vi "64x128OLED_SSD1315YellowBlue.vi"() -> ()   [LabVIEW 2024]
uses:
  Driver/Public/Digital Pull Direction.ctl
  a7562c57-8a3f-42dc-a248-a218528d61d2.vi
  526a81f8-07e3-4dc8-9390-ead75d1578b4.vi
  Public/InitialiseOLED.vi
  Public/GetPicture.vi
  Public/BuildMessagesFromPicture.vi
  Driver/CTIPicoVISA.lvlib
  OLEDI2CMessageGenerator.lvlib
panel:
  in  "Blue 3":string="Blue3"
  in  "Blue 2":string="Blue2"
  in  "Blue 1":string="Blue1"
  in  "Yellow":string="Yellow"
  out "Numeric":i32
  in  "stop":bool
  out "2D Picture":picture
  in  "Grove Connector":enum16{"I2C0", "I2C1"}(ring)
  out "Identity":T1
  out "error out":errorcluster
  in  "Port":refnum<visa-resource-name>="COM7"
  # "https://wiki.seeedstudio.com/Grove-OLED-Yellow&Blue-Display-0.96-SSD1315_V1.0/"
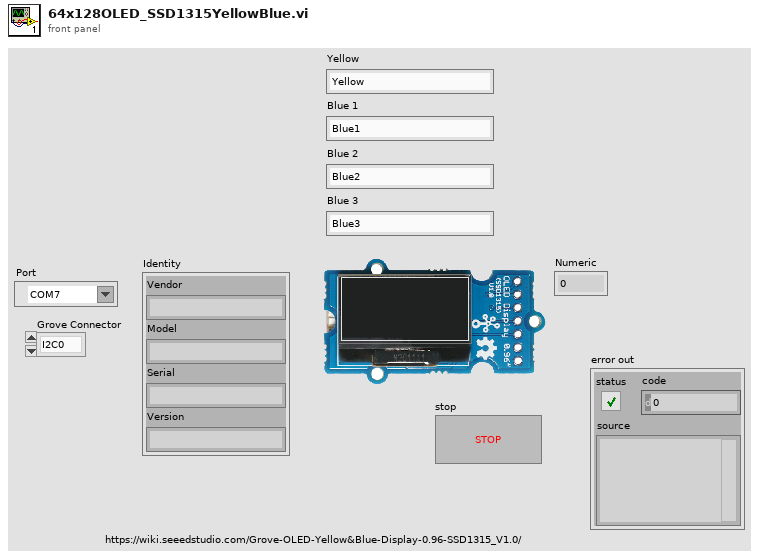
[diagram p1: front panel]
types:
  T1 = cluster{"Vendor":string, "Model":string, "Serial":string, "Version":string}
  T2 = cluster{"Font Name:":string, "Size":i16, "Strikeout?":bool, "Italic?":bool, "Underline?":bool, "Outline?":bool, "Shadow?":bool, "Bold?":bool}
  T3 = typedef "CTIPicoVISA.lvlib/Digital Pull Direction.ctl" = enum16{"None", "Up", "Down", "Both"}
  T4 = enum16{"User-specified Font", "Application Font", "System Font", "Dialog Font"}
  T5 = cluster{"horizontal":enum16{"left", "center", "right"}, "vertical":enum16{"top", "center", "bottom"}}
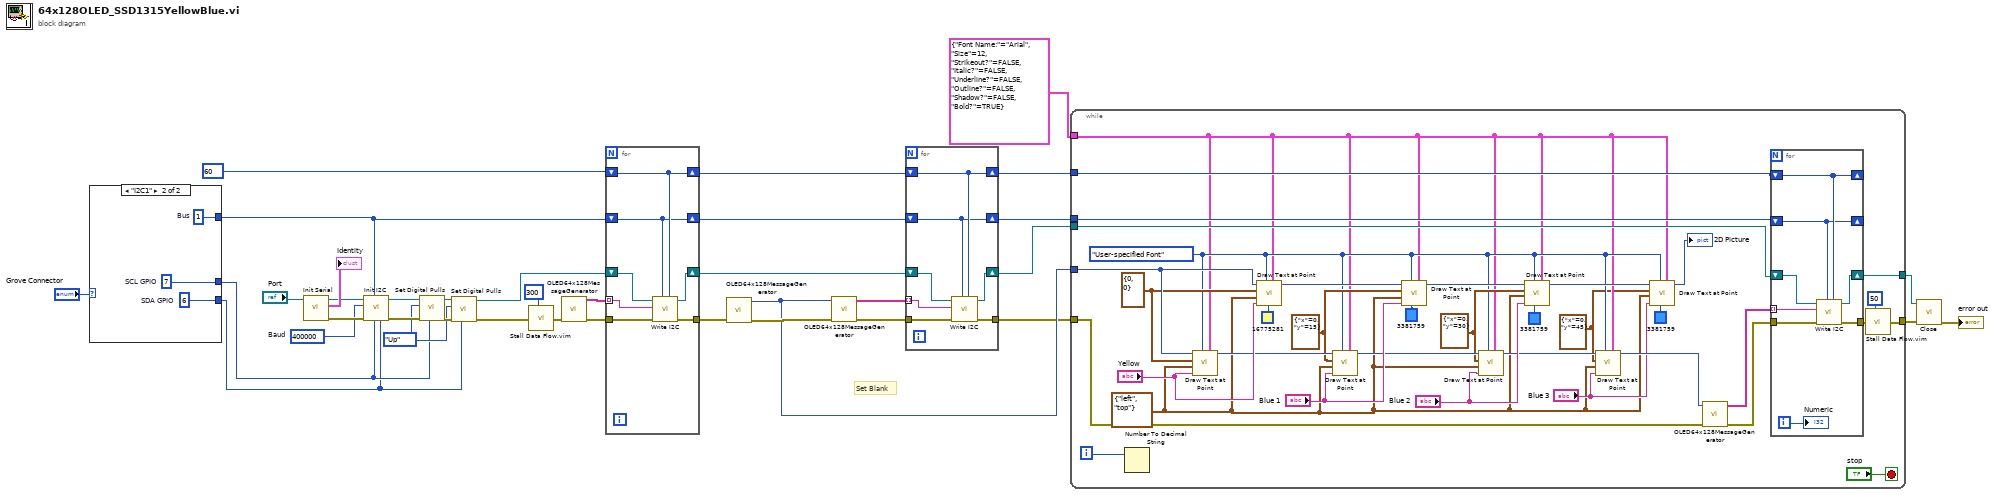
[diagram p0: block diagram]
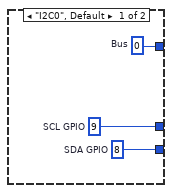
[diagram p2: hidden frame]
diagram:
  w28 = Digital_Pull_Direction."Up" ("Pull")
  w23 = u32 400000  # Baud
  # "Set Blank"
  n1 = case shown="\"I2C1\"" "Grove Connector" {
    tunnel: [w40 w43] -> w15
    tunnel: [w39 w42] -> w14
    tunnel: [w38 w41] -> w21
    frame "I2C0", Default {
      w38 = u8 0  # Bus
      w39 = 8  # SDA GPIO
      w40 = 9  # SCL GPIO
    }
    frame "I2C1" {
      w41 = u8 1  # Bus
      w42 = 6  # SDA GPIO
      w43 = 7  # SCL GPIO
    }
  }
  n2 = call "Init Serial.vi"("VISA resource name in"="Port") -> ("error out"=w24:errorcluster, "Identity"=→"Identity":T1, "VISA resource name Out"=w25:refnum<visa-resource-name>)  [unwired: 8 in]
  n3 = call "Init I2C.vi"("SDA GPIO"=w14, "SCL GPIO"=w15, "Bus"=w21, "error in (no error)"=w24, "Baud"=w23, "VISA resource name in"=w25) -> ("error out"=w31:errorcluster, "VISA resource name"=w32:refnum<visa-resource-name>)  [unwired: 4 in]
  n4 = call "Set Digital Pulls.vi"("GPIO"=w15, "error in (no error)"=w31, "Pull"=w28, "VISA resource name in"=w32) -> ("error out"=w29:errorcluster, "VISA resource name"=w30:refnum<visa-resource-name>)  [unwired: 6 in]
  n5 = call "Set Digital Pulls.vi"("GPIO"=w14, "error in (no error)"=w29, "Pull"=w28, "VISA resource name in"=w30) -> ("error out"=w11:errorcluster, "VISA resource name"=w10:refnum<visa-resource-name>)  [unwired: 6 in]
  n6 = call "Stall Data Flow.vim"("value in"=w11, "milliseconds to wait"=u32 300) -> ("value out"=w26:errorcluster)  [unwired: 1 out]
  n7 = call-poly "OLED64x128MessageGenerator.vi"("error in (no error)"=w26) -> ("error out"=w22:errorcluster, "Messages"=w33:string[])  [unwired: 9 in]
  n8 = for {
    tunnel: w33 -> [w48] mode=indexing
    tunnel: w22 -> [w50]
    tunnel: [w47] -> w19
    shift-right: [w46] -> w5
    shift-left: w10 -> [w49]
    shift-right: [w45] -> w6
    shift-left: u8 60 ("Address") -> [w45]
    shift-right: [w44] -> w4
    shift-left: w21 -> [w44]
    n9 = call "Write I2C.vi"("Address"=w45, "Bus"=w44, "error in (no error)"=w50, "Data"=w48, "VISA resource name in"=w49) -> ("error out"=w47:errorcluster, "VISA resource name"=w46:refnum<visa-resource-name>)  [unwired: 5 in]
  }
  n10 = call-poly "OLED64x128MessageGenerator.vi"("error in (no error)"=w19) -> ("error out"=w13:errorcluster, "2D Picture"=w12:picture)  [unwired: 9 in]
  n11 = call-poly "OLED64x128MessageGenerator.vi"("error in (no error)"=w13, "2D Picture"=w12) -> ("error out"=w9:errorcluster, "Messages"=w8:string[])  [unwired: 8 in]
  n12 = for {
    tunnel: w8 -> [w55] mode=indexing
    tunnel: w9 -> [w57]
    tunnel: [w54] -> w7
    shift-right: [w53] -> w3
    shift-left: w5 -> [w56]
    shift-right: [w52] -> w1
    shift-left: w6 -> [w52]
    shift-right: [w51] -> w2
    shift-left: w4 -> [w51]
    n13 = call "Write I2C.vi"("Address"=w52, "Bus"=w51, "error in (no error)"=w57, "Data"=w55, "VISA resource name in"=w56) -> ("error out"=w54:errorcluster, "VISA resource name"=w53:refnum<visa-resource-name>)  [unwired: 5 in]
  }
  n14 = while {
    tunnel: w12 -> [w80]
    tunnel: w7 -> [w93]
    tunnel: w1 -> [w92]
    tunnel: w2 -> [w91]
    tunnel: w3 -> [w90]
    tunnel: [w87] -> w17
    tunnel: [w83] -> w18
    tunnel: T2 {"Font Name:"="Arial", "Size"=12, "Strikeout?"=FALSE, "Italic?"=FALSE, "Underline?"=FALSE, "Outline?"=FALSE, "Shadow?"=FALSE, "Bold?"=TRUE} ("[user-specified font]") -> [w59]
    i -> [w85]
    stop <- "stop" stop-if-true
    w58 = cluster{"x":i16, "y":i16} {"x"=0, "y"=45} ("origin")
    w68 = cluster{"x":i16, "y":i16} {"x"=0, "y"=30} ("origin")
    w73 = cluster{"x":i16, "y":i16} {"x"=0, "y"=15} ("origin")
    w60 = T4."User-specified Font" ("desired font(Application)")
    w61 = T5 {"horizontal"=enum."left", "vertical"=enum."top"} ("alignment(left, top)")
    w78 = cluster{"x":i16, "y":i16} {"x"=0, "y"=0} ("origin")
    n15 = Number To Decimal String(number=w85) -> ()  [unwired: 1 in, 1 out]
    n16 = call <vilib>:"Draw Text at Point.vi"("[user-specified font]"=w59, "desired font(Application)"=w60, "text"="Yellow", "alignment(left, top)"=w61, "origin"=w78, "picture"=w80) -> ("new picture"=w75:picture)  [unwired: 4 in, 1 out]
    n17 = call <vilib>:"Draw Text at Point.vi"("[user-specified font]"=w59, "text color(black)"=u32 16775281 ("text color"), "desired font(Application)"=w60, "text"="Yellow", "alignment(left, top)"=w61, "origin"=w78, "picture"=w80) -> ("new picture"=w77:picture)  [unwired: 3 in, 1 out]
    n18 = call <vilib>:"Draw Text at Point.vi"("[user-specified font]"=w59, "desired font(Application)"=w60, "text"="Blue 1", "alignment(left, top)"=w61, "origin"=w73, "picture"=w75) -> ("new picture"=w72:picture)  [unwired: 4 in, 1 out]
    n19 = call <vilib>:"Draw Text at Point.vi"("[user-specified font]"=w59, "text color(black)"=u32 3381759, "desired font(Application)"=w60, "text"="Blue 1", "alignment(left, top)"=w61, "origin"=w73, "picture"=w77) -> ("new picture"=w69:picture)  [unwired: 3 in, 1 out]
    n20 = call <vilib>:"Draw Text at Point.vi"("[user-specified font]"=w59, "desired font(Application)"=w60, "text"="Blue 2", "alignment(left, top)"=w61, "origin"=w68, "picture"=w72) -> ("new picture"=w67:picture)  [unwired: 4 in, 1 out]
    n21 = call <vilib>:"Draw Text at Point.vi"("[user-specified font]"=w59, "text color(black)"=u32 3381759, "desired font(Application)"=w60, "text"="Blue 2", "alignment(left, top)"=w61, "origin"=w68, "picture"=w69) -> ("new picture"=w65:picture)  [unwired: 3 in, 1 out]
    n22 = call <vilib>:"Draw Text at Point.vi"("[user-specified font]"=w59, "desired font(Application)"=w60, "text"="Blue 3", "alignment(left, top)"=w61, "origin"=w58, "picture"=w67) -> ("new picture"=w66:picture)  [unwired: 4 in, 1 out]
    n23 = call <vilib>:"Draw Text at Point.vi"("[user-specified font]"=w59, "text color(black)"=u32 3381759, "desired font(Application)"=w60, "text"="Blue 3", "alignment(left, top)"=w61, "origin"=w58, "picture"=w65) -> ("new picture"=→"2D Picture":picture)  [unwired: 3 in, 1 out]
    n24 = call-poly "OLED64x128MessageGenerator.vi"("error in (no error)"=w93, "2D Picture"=w66) -> ("error out"=w89:errorcluster, "Messages"=w88:string[])  [unwired: 8 in]
    n25 = for {
      tunnel: w88 -> [w99] mode=indexing
      tunnel: w89 -> [w101]
      tunnel: [w98] -> w84
      shift-right: [w97] -> w87
      shift-left: w90 -> [w100]
      shift-right: [w96] -> _
      shift-left: w92 -> [w96]
      shift-right: [w95] -> _
      shift-left: w91 -> [w95]
      i -> [w94]
      n26 = call "Write I2C.vi"("Address"=w96, "Bus"=w95, "error in (no error)"=w101, "Data"=w99, "VISA resource name in"=w100) -> ("error out"=w98:errorcluster, "VISA resource name"=w97:refnum<visa-resource-name>)  [unwired: 5 in]
      "Numeric" <- w94
    }
    n27 = call "Stall Data Flow.vim"("value in"=w84, "milliseconds to wait"=u32 50) -> ("value out"=w83:errorcluster)  [unwired: 1 out]
  }
  n28 = call "Close.vi"("error in (no error)"=w18, "VISA resource name in"=w17) -> ("error out"=→"error out":errorcluster)  [unwired: 9 in]
